vi "Get Cookie Name.vi"(8 "error in (no error)":errorcluster, 11 "Session in":refnum<class "Session.lvclass">) -> (0 "error out":errorcluster, 2 "Cookie Name":string, 3 "Session out":refnum<class "Session.lvclass">)   [LabVIEW 2020, in "HTTP Server.lvlib" / "Session.lvclass"]
uses:
  Session.lvclass
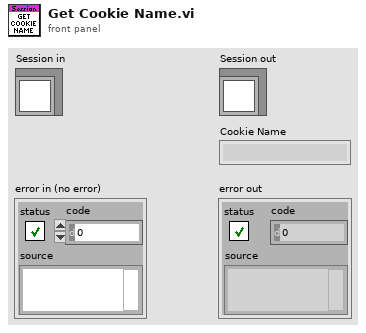
[diagram p1: front panel]
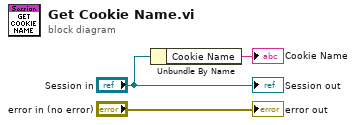
[diagram p0: block diagram]
diagram:
  n1 = Unbundle By Name("Session in") -> ("Cookie Name"=→"Cookie Name":string)
  "error out" <- "error in (no error)"
  "Session out" <- "Session in"
